vi "convertmm-to-ps.vi"(1 "mm":dbl, 2 "Real zero":dbl) -> (0 "ps":dbl)   [LabVIEW 2020]
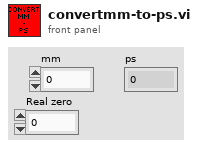
[diagram p1: front panel]
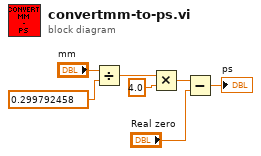
[diagram p0: block diagram]
diagram:
  n1 = Divide(x="mm", y=0.299792458) -> (x/y=w6:dbl)
  n2 = Multiply(x=w6, y=4.0) -> (x*y=w3:dbl)
  n3 = Subtract(x=w3, y="Real zero") -> (x-y=→"ps":dbl)
